vi "F Dwf Digital Uart Tx.vi"(8 "error in (no error)":errorcluster, 9 "cTx":i32, 10 "szTx":string, 11 "hdwf":i32) -> (0 "error out":errorcluster, 2 "szTx out":string, 3 "function return":i32)   [LabVIEW 2021, in "Olasdwf.lvlib"]
doc: "DWFAPI int FDwfDigitalUartTx(HDWF hdwf, char *szTx, int cTx);"
uses:
  Olasdwf.lvlib
  Windows/System32/dwf.dll
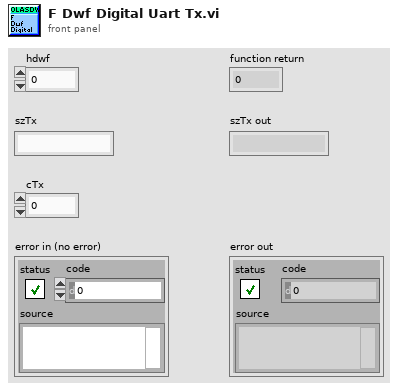
[diagram p1: front panel]
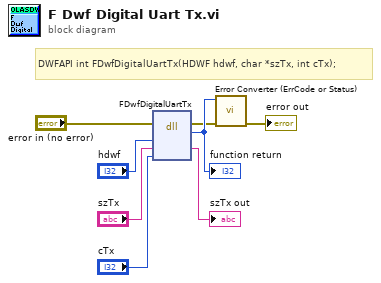
[diagram p0: block diagram]
diagram:
  # "DWFAPI int FDwfDigitalUartTx(HDWF hdwf, char *szTx, int cTx);"
  n1 = dll-call lib="/Windows/System32/dwf.*" fn="FDwfDigitalUartTx"(error in="error in (no error)", "hdwf"="hdwf", "szTx"="szTx", "cTx"="cTx") -> (error out=w2:errorcluster, w8:i32, "szTx"=→"szTx out":string)  [unwired: 4 in, 1 out]
  "function return" <- w8
  n2 = call "Error Converter (ErrCode or Status).vi"("error in (no error)"=w2, "error code"=w8) -> ("error out"=→"error out":errorcluster)  [unwired: 9 in]
